vi "OnLoad - Add Missing CD Ports for unreferenced NI-XNET Ports.vi"(8 "error in (no error)":errorcluster, 11 "Device Item Ref in in":T1 format="%.0x") -> (0 "error out":errorcluster, 3 "Device Item Ref out":T1 format="%.0x")   [LabVIEW 2017, in "NI-XNET Monitor System Explorer.lvlib"]
uses:
  NI-XNET Monitor System Explorer.lvlib
  <vilib>/NI Veristand/Custom Device API/Custom Device Item Ref.ctl
  <vilib>/NI Veristand/Custom Device API/Custom Device API.lvlib
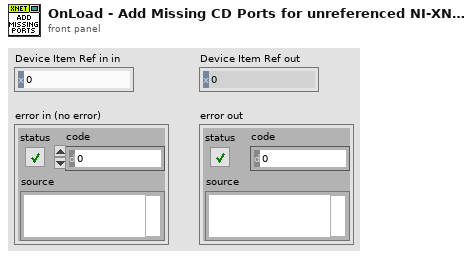
[diagram p1: front panel]
types:
  T1 = typedef "Custom Device API.lvlib/Custom Device Item Ref.ctl" = u64
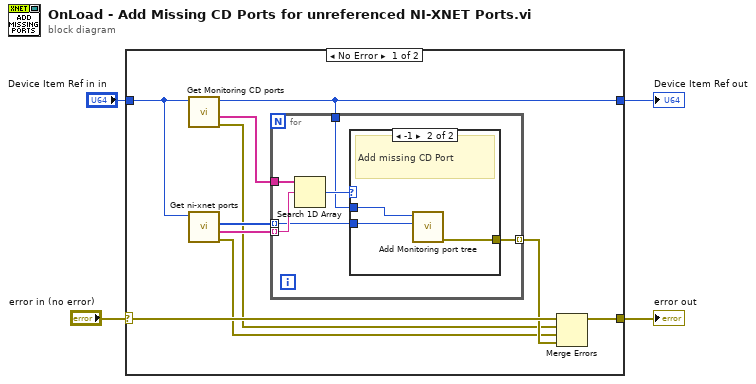
[diagram p0: block diagram]
diagram:
  n1 = case shown="No Error" "error in (no error)" {
    selector: "error in (no error)" -> [w14 w25]
    tunnel: [w13 w25] -> w2
    tunnel: "Device Item Ref in in" -> [w7 w24]
    tunnel: [w5 w24] -> w4
    frame No Error {
      n2 = call "Get Monitoring CD ports.vi"("Device Item Ref in"=w7) -> ("Error Out"=w8:errorcluster, "Referenced NI-XNET Port Item Paths"=w6:string[], "Device Item Ref out"=w5:T1)  [unwired: 7 in, 1 out]
      n3 = call "Get ni-xnet ports.vi"("Device Item Ref in"=w7) -> ("Error Out"=w9:errorcluster, "NI-XNET Port Item Paths"=w10:string[], "NI-XNET Port Refs"=w11:T1[])  [unwired: 7 in, 1 out]
      n4 = for {
        tunnel: w10 -> [w19] mode=indexing
        tunnel: w11 -> [w17] mode=indexing
        tunnel: w6 -> [w20]
        tunnel: [w16] -> w12 mode=indexing
        tunnel: w5 -> [w15]
        n5 = Search 1D Array(1D array=w20, element=w19) -> (index of element=w18:i32)  [unwired: 1 in]
        n6 = case shown="-1" w18 {
          tunnel: w17 -> [_ w21]
          tunnel: [_ w22] -> w16
          tunnel: w15 -> [_ w23]
          frame Default {
            # "do nothing"
          }
          frame -1 {
            # "Add missing CD Port"
            n7 = call "Add Monitoring port tree.vi"("NI-XNET Port (Item Ref)"=w21, "Device Item Ref in"=w23) -> ("Error Out"=w22:errorcluster)  [unwired: 8 in, 1 out]
          }
        }
      }
      n8 = Merge Errors(w14, w8, w9, w12) -> (w13:errorcluster)
    }
    frame Error {
    }
  }
  "Device Item Ref out" <- w4
  "error out" <- w2
